vi "writeCTOarrays.vi"(0 "System no.":i32=1 min=1 max=4 step=1, 5 "CTOparamValArray":string[](array[string]), 7 "triggIdxArray":string[](array[string]), 9 "CTO parameter ID":i32[](array[numeric])=[2, 3, 1, 10, 9], 11 "error in":errorcluster) -> (8 "error out":errorcluster)   [LabVIEW 2015]
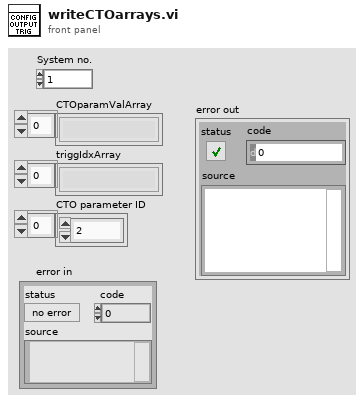
[diagram p1: front panel]
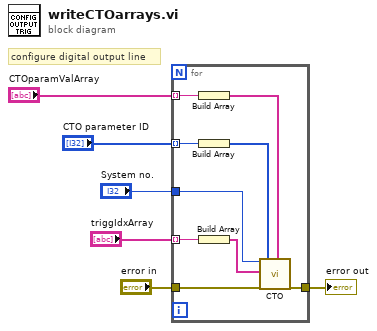
[diagram p0: block diagram]
diagram:
  # "configure digital output line"
  n1 = for {
    tunnel: "CTOparamValArray" -> [w15] mode=indexing
    tunnel: "triggIdxArray" -> [w14] mode=indexing
    tunnel: "CTO parameter ID" -> [w13] mode=indexing
    tunnel: [w9] -> w3
    tunnel: "error in" -> [w8]
    tunnel: "System no." -> [w7]
    n2 = Build Array(w15) -> (w11:string[])
    n3 = Build Array(w13) -> (w12:i32[])
    n4 = Build Array(w14) -> (w10:string[])
    n5 = call "CTO.vi"("System no."=w7, "TriggerOut to set"=w10, "error in"=w8, "CTO parameter ID"=w12, "Parameter value"=w11) -> ("error out"=w9:errorcluster)  [unwired: 13 in, 1 out]
  }
  "error out" <- w3
